vi "FMPM-Erzeugung.vi"() -> ()   [LabVIEW 2017]
uses:
  <vilib>/sound2/lvsound2.llb/Sampling Mode.ctl
  <vilib>/sound2/lvsound2.llb/Sound Data Format.ctl
  <vilib>/Utility/error.llb/DialogType.ctl
  <vilib>/Analysis/2dsp.llb/Integral Method.ctl
  <vilib>/express/express analysis/Spectral/Block/exnSpectralBlock spectral measurements RMS poly.vi
  <vilib>/express/express analysis/Spectral/Block/exnSpectralBlock spectral measurements RMS WFM.vi
  <vilib>/sound2/lvsound2.llb/Sound Output Write (DBL Single).vi
  <vilib>/express/express analysis/Spectral/XNode/ExpressSpectralMeasurementsBlockNode.xnode
  <vilib>/Analysis/NI_AALPro.lvlib
panel:
  in  "Modulationsart":enum16{"PM", "FM"}(ring)=enum."FM"
  in  "k":dbl=0.005
  in  "stop":bool
  out "Ausgang: Zeitbild":dbl[](graph)
  out "Ausgang: Frequenzbild":cluster{"f0":dbl, "df":dbl, "magnitude":dbl[]}(graph)={"f0"=0.0, "df"=2.2675736961451248e-05, "magnitude"=array[22050 elements]}
  in  "Signalamplitude 2":dbl=6.0
  in  "Signalamplitude 1":dbl=3.0
  in  "Signalfrequenz 2":dbl=1000.0
  in  "Signalfrequenz 1":dbl=700.0
  in  "Trägerfrequenz":dbl=10000.0
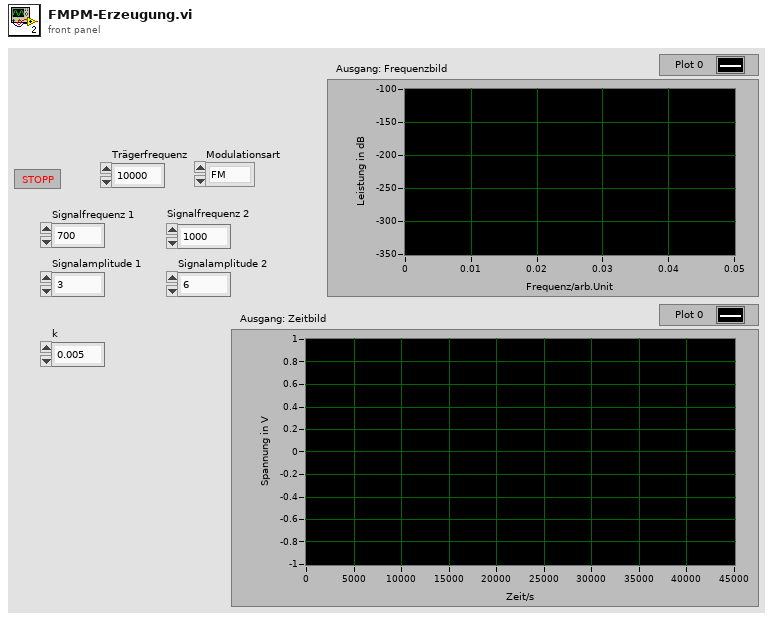
[diagram p1: front panel]
types:
  T1 = typedef "Sound Data Format.ctl" = cluster{"sample rate (S/s)":dbl, "number of channels":i32, "bits per sample":i32}
  T2 = cluster{"averaging mode":u16, "weighting mode":u16, "number of averages":u32}
  T3 = cluster{"dB On (F)":bool, "unwrap phase (F)":bool, "convert to degree (F)":bool}
  T4 = typedef "DialogType.ctl" = u16
  T5 = typedef "Sampling Mode.ctl" = i32
  T6 = typedef "NI_AALPro.lvlib/Integral Method.ctl" = i32
  T7 = typedef "Sound Output Task ID.ctl" = u32
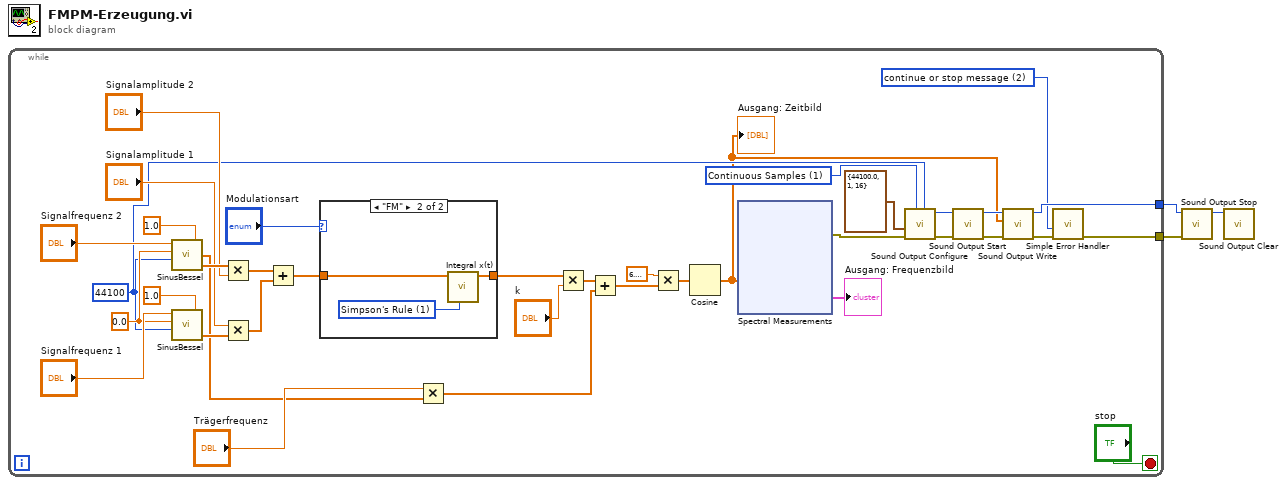
[diagram p0: block diagram]
diagram:
  n1 = while {
    tunnel: [w22] -> w2
    tunnel: [w24] -> w1
    stop <- "stop" stop-if-true
    w21 = T4 2 items=["no dialog", "OK message", "continue or stop message", "OK message + warnings", "continue/stop + warnings"] ("type of dialog (OK msg:1)")
    w13 = 44100 ("number of samples/ch")
    w30 = T5 1 items=["Finite Samples", "Continuous Samples"] ("sample mode")
    w37 = 0.0 ("Phase phi")
    n2 = call "SinusBessel.vi"("Amplitude A"=1.0, "Zahl der Punkte N"=w13, "Phase phi"=w37, "Frequenz f"="Signalfrequenz 2") -> ("y"=w38:dbl[], "Zeit t"=w6:dbl[])  [unwired: 1 in]
    n3 = call "SinusBessel.vi"("Amplitude A"=1.0, "Zahl der Punkte N"=w13, "Phase phi"=w37, "Frequenz f"="Signalfrequenz 1") -> ("y"=w35:dbl[])  [unwired: 1 in, 1 out]
    n4 = Multiply(x=w38, y="Signalamplitude 2") -> (x*y=w31:dbl[])
    n5 = Multiply(x="Signalamplitude 1", y=w35) -> (x*y=w33:dbl[])
    n6 = Add(x=w31, y=w33) -> (x+y=w11:dbl[])
    n7 = case shown="\"FM\"" "Modulationsart" {
      tunnel: w11 -> [w41 w44]
      tunnel: [w41 w43] -> w10
      frame "PM" {
      }
      frame "FM" {
        w42 = T6 1 items=["Trapezoidal Rule", "Simpson's Rule", "Simpson's 3/8 Rule", "Bode Rule"] ("integration method")
        n8 = call <vilib>:"Integral x(t).vi"("integration method"=w42, "X"=w44) -> ("Integral X"=w43:dbl[])  [unwired: 8 in, 1 out]
      }
    }
    n9 = Multiply(x="Trägerfrequenz", y=w6) -> (x*y=w9:dbl[])
    n10 = Multiply(x=w10, y="k") -> (x*y=w15:dbl[])
    n11 = Add(x=w15, y=w9) -> (x+y=w8:dbl[])
    n12 = Multiply(x=6.283185307179586, y=w8) -> (x*y=w5:dbl[])
    n13 = Cosine(x=w5) -> (cos(x)=w4:dbl[])
    "Ausgang: Zeitbild" <- w4
    n14 = xnode "Spectral Measurements"("Signals"=w4) -> ("FFT - (RMS)"=→"Ausgang: Frequenzbild":cluster{"f0":dbl, "df":dbl, "magnitude":dbl[]}, "error out"=w17:errorcluster)  [unwired: 1 in, 1 out]
    n15 = call <vilib>:"Sound Output Configure.vi"("number of samples/ch"=w13, "sample mode"=w30, "error in (no error)"=w17, "sound format"=T1 {"sample rate (S/s)"=44100.0, "number of channels"=1, "bits per sample"=16}) -> ("error out"=w29:errorcluster, "task ID"=w26:T7)  [unwired: 6 in]
    n16 = call <vilib>:"Sound Output Start.vi"("error in (no error)"=w29, "task ID"=w26) -> ("error out"=w28:errorcluster, "task ID out"=w25:T7)  [unwired: 8 in]
    n17 = call-poly <vilib>:"Sound Output Write.vi"("error in (no error)"=w28, "data"=w4, "task ID"=w25) -> ("error out"=w23:errorcluster, "task ID out"=w24:T7)  [unwired: 7 in]
    n18 = call <vilib>:"Simple Error Handler.vi"("type of dialog (OK msg:1)"=w21, "error in (no error)"=w23) -> ("error out"=w22:errorcluster)  [unwired: 3 in, 4 out]
  }
  n19 = call <vilib>:"Sound Output Stop.vi"("error in (no error)"=w2, "task ID"=w1) -> ("task ID out"=w3:T7)  [unwired: 8 in, 1 out]
  n20 = call <vilib>:"Sound Output Clear.vi"("task ID"=w3) -> ()  [unwired: 10 in, 1 out]
